vi "TIME FGV.vi"(10 "Enum":enum16{"Elapsed?", "SetTime"}(ring), 11 "Time in seconds":u32) -> (3 "Time Elapsed?":bool)   [LabVIEW 2020]
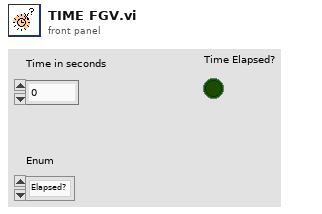
[diagram p1: front panel]
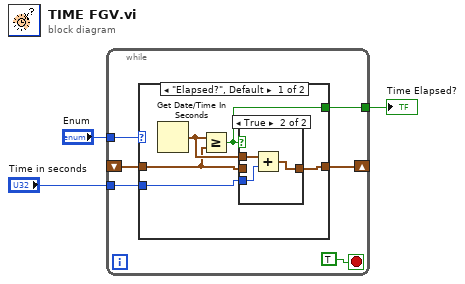
[diagram p0: block diagram]
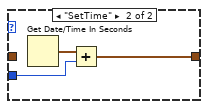
[diagram p3: hidden frame]
diagram:
  n1 = while {
    tunnel: "Enum" -> [w9]
    tunnel: "Time in seconds" -> [w8]
    shift-right: [w6] -> _
    shift-left: _ -> [w7]
    tunnel: [w5] -> w1
    stop <- TRUE stop-if-true
    n2 = case shown="\"Elapsed?\", Default" w9 {
      tunnel: w8 -> [w12 w20]
      tunnel: w7 -> [w10 _]
      tunnel: [w11 w19] -> w6
      tunnel: [w14 _] -> w5
      frame "Elapsed?", Default {
        n3 = Get Date/Time In Seconds() -> (seconds since 1Jan1904=w13:timestamp)
        n4 = Greater Or Equal?(x=w13, y=w10) -> (x >= y?=w14:bool)
        n5 = case shown="True" w14 {
          tunnel: w13 -> [_ w18]
          tunnel: w12 -> [_ w17]
          tunnel: [w15 w16] -> w11
          tunnel: w10 -> [w15 _]
          frame False {
          }
          frame True {
            n6 = Add(x=w18, y=w17) -> (x+y=w16:timestamp)
          }
        }
      }
      frame "SetTime" {
        n7 = Get Date/Time In Seconds() -> (seconds since 1Jan1904=w21:timestamp)
        n8 = Add(x=w21, y=w20) -> (x+y=w19:timestamp)
      }
    }
  }
  "Time Elapsed?" <- w1
